vi "LJstreamM add data to file.vi"(4 "Scan Rate":dbl=50.0 format="%.2f", 6 "Time":dbl format="%.2f", 8 "Disable Scaling":bool, 9 "Scaled Data":dbl[][](array[numeric]) format="%.3f", 10 "Voltages":dbl[][](array[numeric]) format="%.3f", 11 "file path":path) -> (0 "error":bool)   [LabVIEW 2025]
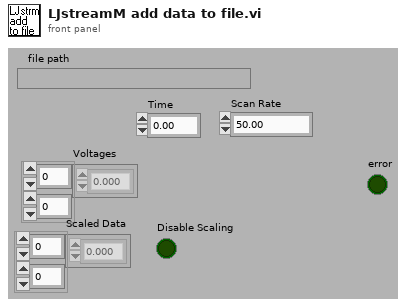
[diagram p1: front panel]
types:
  T1 = enum16{"open", "open or create", "create or replace", "create", "open (read only)"}
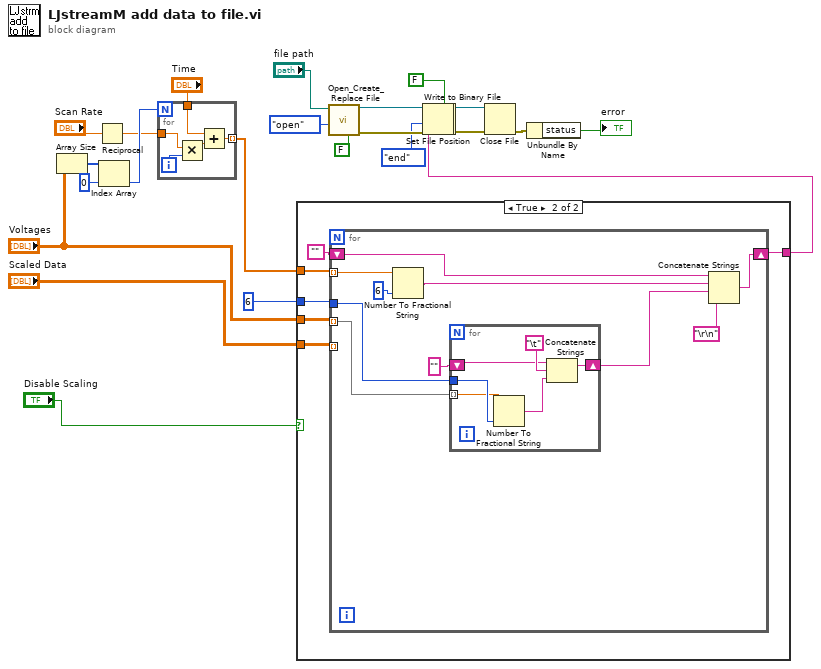
[diagram p0: block diagram]
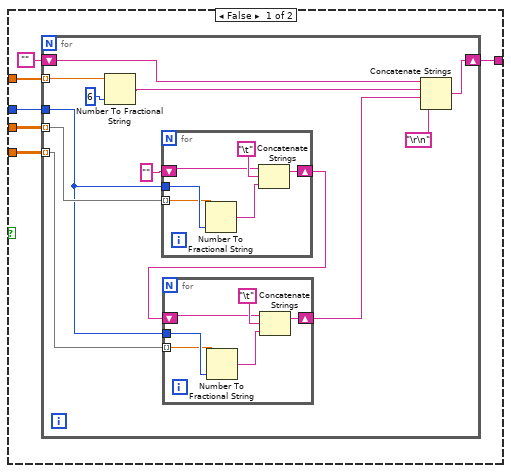
[diagram p2: hidden frame]
diagram:
  n1 = Array Size(array="Voltages") -> (size(s)=w15:i32[])
  n2 = Reciprocal(x="Scan Rate") -> (1/x=w10:dbl)
  n3 = Index Array(array=w15, index=0 ("Index")) -> (element=w13:i32)
  n4 = for {
    N: w13 -> [_]
    tunnel: "Time" -> [w30]
    tunnel: w10 -> [w26]
    tunnel: [w29] -> w9 mode=indexing
    i -> [w27]
    n5 = Multiply(x=w26, y=w27) -> (x*y=w28:dbl)
    n6 = Add(x=w30, y=w28) -> (x+y=w29:dbl)
  }
  n7 = case shown="True" "Disable Scaling" {
    tunnel: w9 -> [w36 w62]
    tunnel: "Voltages" -> [w35 w64]
    tunnel: "Scaled Data" -> [w34 w65]
    tunnel: [w33 w61] -> w6
    tunnel: i16 6 ("precision (6)") -> [w32 w63]
    frame False {
      n8 = for {
        shift-right: [w44] -> w33
        shift-left: "" -> [w45]
        tunnel: w36 -> [w47] mode=indexing
        tunnel: w35 -> [w42] mode=indexing
        tunnel: w34 -> [w37] mode=indexing
        tunnel: w32 -> [w38]
        n9 = Number To Fractional String(number=w47, precision (6)=i16 6) -> (F-format string=w46:string)  [unwired: 2 in]
        n10 = for {
          shift-right: [w58] -> w40
          shift-left: "" -> [w59]
          tunnel: w38 -> [w56]
          tunnel: w42 -> [w55] mode=indexing
          n11 = Number To Fractional String(number=w55, precision (6)=w56) -> (F-format string=w57:string)  [unwired: 2 in]
          n12 = Concatenate Strings(w59, "\t", w57) -> (w58:string)
        }
        n13 = for {
          shift-right: [w52] -> w39
          shift-left: w40 -> [w53]
          tunnel: w38 -> [w50]
          tunnel: w37 -> [w49] mode=indexing
          n14 = Number To Fractional String(number=w49, precision (6)=w50) -> (F-format string=w51:string)  [unwired: 2 in]
          n15 = Concatenate Strings(w53, "\t", w51) -> (w52:string)
        }
        n16 = Concatenate Strings(w45, w46, w39, "\r\n") -> (w44:string)
      }
    }
    frame True {
      n17 = for {
        shift-right: [w72] -> w61
        shift-left: "" -> [w73]
        tunnel: w62 -> [w75] mode=indexing
        tunnel: w64 -> [w70] mode=indexing
        tunnel: w65 -> [_] mode=indexing
        tunnel: w63 -> [w68]
        n18 = Number To Fractional String(number=w75, precision (6)=i16 6) -> (F-format string=w74:string)  [unwired: 2 in]
        n19 = for {
          shift-right: [w80] -> w67
          shift-left: "" -> [w81]
          tunnel: w68 -> [w78]
          tunnel: w70 -> [w77] mode=indexing
          n20 = Number To Fractional String(number=w77, precision (6)=w78) -> (F-format string=w79:string)  [unwired: 2 in]
          n21 = Concatenate Strings(w81, "\t", w79) -> (w80:string)
        }
        n22 = Concatenate Strings(w73, w74, w67, "\r\n") -> (w72:string)
      }
    }
  }
  n23 = call <vilib>:"Open_Create_Replace File.vi"("advisory dialog? (display:T)"=FALSE, "function (open:0)"=T1."open", "file path"="file path") -> ("error out"=w22:errorcluster, "refnum"=w23:refnum<file>)  [unwired: 5 in, 2 out]
  n24 = Set File Position(refnum=w23, from (0:start)=enum16{"start", "end", "current"}."end" ("pos mode (0:2)"), error in=w22) -> (refnum out=w3:refnum<file>, error out=w2:errorcluster)  [unwired: 1 in]
  n25 = Write to Binary File(file (use dialog)=w3, data=w6, error in=w2, 5:FALSE ("prepend array or string size? (T)")) -> (refnum out=w25:refnum<file>, error out=w24:errorcluster)  [unwired: 2 in, 1 out]
  n26 = Close File(refnum=w25, error in=w24) -> (error out=w17:errorcluster)  [unwired: 1 out]
  n27 = Unbundle By Name(w17) -> ("status"=→"error":bool)
